vi "Get or Add Stylesheet.vi"(8 "error in":errorcluster, 11 "SpreadsheetDoc in":refnum<k24>) -> (0 "error out":errorcluster, 2 "Stylesheet":refnum<k24>, 3 "SpreadsheetDoc out":refnum<k24>)   [LabVIEW 2021, in "Open Xml.lvlib"]
uses:
  Open Xml.lvlib
  D:/git/Open-Xml-LabVIEW/dll/DocumentFormat.OpenXml.dll
  dll/DocumentFormat.OpenXml.dll
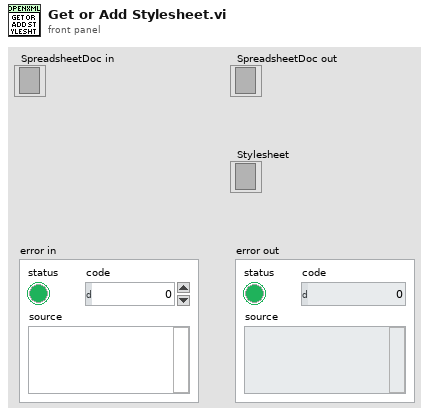
[diagram p1: front panel]
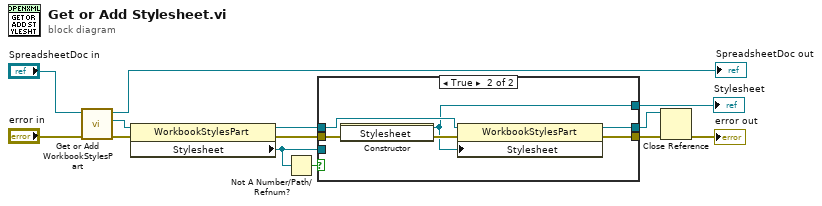
[diagram p0: block diagram]
diagram:
  n1 = call "Get or Add WorkbookStylesPart.vi"("error in"="error in", "SpreadsheetDoc in"="SpreadsheetDoc in") -> ("error out"=w10:errorcluster, "WorkbookStylesPart"=w9:refnum<k24>, "SpreadsheetDoc out"=→"SpreadsheetDoc out":refnum<k24>)  [unwired: 7 in]
  n2 = property class="WorkbookStylesPart"(reference=w9, error in=w10) -> (reference out=w2:refnum<k24>, error out=w4:errorcluster, "Stylesheet"=w5:refnum<k24>)
  n3 = Not A Number/Path/Refnum?(number/path/refnum=w5) -> (NaN/Path/Refnum?=w6:bool)
  n4 = case shown="True" w6 {
    tunnel: w5 -> [w14 _]
    tunnel: [w14 w18] -> w7
    tunnel: w4 -> [w15 w22]
    tunnel: [w15 w20] -> w3
    tunnel: w2 -> [w16 w19]
    tunnel: [w16 w17] -> w1
    frame False {
    }
    frame True {
      n5 = constructor class="Stylesheet"(error in=w22) -> (reference out=w18:refnum<k24>, error out=w21:errorcluster)  [unwired: 2 in, 1 out]
      n6 = property class="WorkbookStylesPart"(reference=w19, error in=w21, "Stylesheet"=w18) -> (reference out=w17:refnum<k24>, error out=w20:errorcluster)
    }
  }
  "Stylesheet" <- w7
  n7 = Close Reference(reference=w1, error in (no error)=w3) -> (error out=→"error out":errorcluster)
